vi "Create Header (SubVI).vi"(9 "Frequencies":dbl[](array[numeric]), 10 "Measurement Information":string, 11 "current time":timestamp) -> (2 "Header":string)   [LabVIEW 2017]
uses:
  GlobalVariables/Delimiter.vi
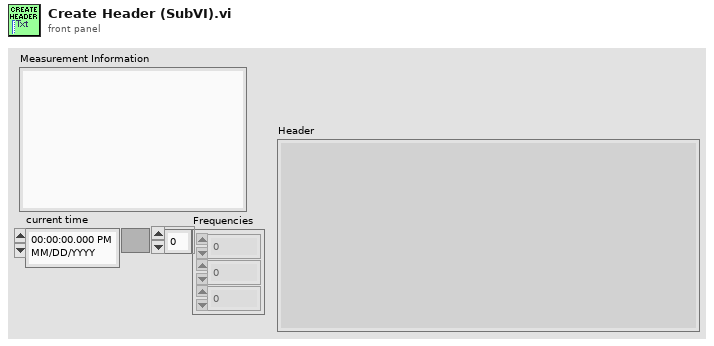
[diagram p1: front panel]
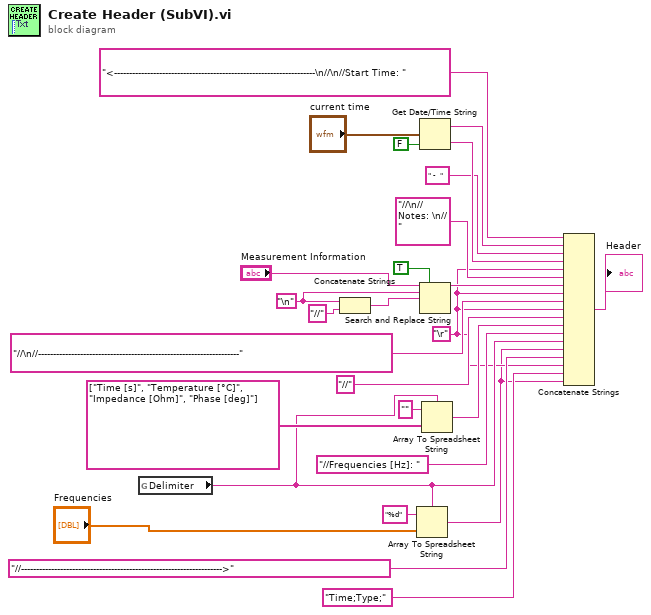
[diagram p0: block diagram]
diagram:
  w18 = "\n"
  w3 = "\r"
  n1 = global read "Delimiter.vi" "Delimiter"() -> (w4:string)
  n2 = Concatenate Strings(w18, "//" ("replace string (\"\")")) -> (w16:string)
  n3 = Array To Spreadsheet String(delimiter (Tab)=w4, array="Frequencies", 3:"%d" ("format string")) -> (spreadsheet string=w1:string)
  n4 = Get Date/Time String(seconds (now)="current time", want seconds? (F)=FALSE) -> (date string=w24:string, time string=w25:string)  [unwired: 1 in]
  n5 = Search and Replace String(replace all?=TRUE ("replace all? (F)"), input string="Measurement Information", search string=w18, replace string=w16) -> (result string=w14:string)  [unwired: 4 in, 3 out]
  n6 = Array To Spreadsheet String(delimiter (Tab)=w4, array=string[] ["Time [s]", "Temperature [°C]", "Impedance [Ohm]", "Phase [deg]"], 3:"" ("format string")) -> (spreadsheet string=w9:string)
  n7 = Concatenate Strings("<-------------------------------------------------------------------\n//\n//Start Time: " ("string"), w24, " -  " ("string"), w25, w3, "//\n//Notes: \n//" ("string"), w14, w3, "//\n//-------------------------------------------------------------------" ("string"), w3, "//" ("string"), w9, "//Frequencies [Hz]: " ("string"), w4, w1, "//------------------------------------------------------------------->" ("string"), w3, "Time;Type;" ("string"), w1) -> (→"Header":string)
